vi "RSNRPZ Read Measurement.vi"(8 "error in (no error)":errorcluster, 9 "Timeout (5000 ms)":i32=5000, 10 "Channel (1)":i32=1, 11 "VISA session":refnum<visa-resource-name>) -> (0 "error out":errorcluster, 2 "Measurement":dbl format="%.3p", 3 "dup VISA session":refnum<visa-resource-name>)   [LabVIEW 2014]
doc: "This VI initiates an acquisition on the channels that you specifies in channel parameter. It then waits for the acquisition to complete, and returns the measurement for the channel you specify."
uses:
  rsnrpz_32.dll
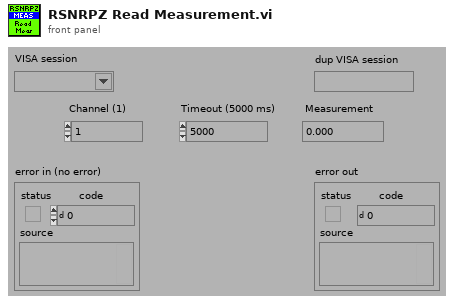
[diagram p1: front panel]
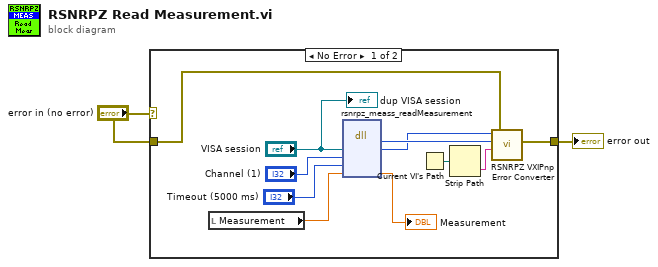
[diagram p0: block diagram]
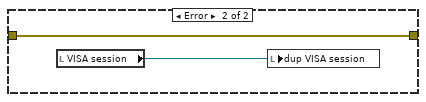
[diagram p2: hidden frame]
diagram:
  n1 = case shown="No Error" "error in (no error)" {
    tunnel: "error in (no error)" -> [w5 w15]
    tunnel: [w6 w15] -> w1
    frame No Error {
      n2 = local read "Measurement"() -> (w9:dbl)
      n3 = dll-call lib="rsnrpz_32.dll" fn="rsnrpz_meass_readMeasurement"("Instrument Handle"="VISA session", "Channel"="Channel (1)", "Timeout (ms)"="Timeout (5000 ms)", "Measurement"=w9) -> ("Status"=w12:i32, "Instrument Handle"=w7:u32, "Measurement"=→"Measurement":dbl)  [unwired: 5 in, 2 out]
      n4 = Current VI's Path() -> (path=w4:path)
      n5 = Strip Path(path=w4) -> (name=w3:string)  [unwired: 1 out]
      n6 = call "RSNRPZ VXIPnp Error Converter.vi"("error in (no error)"=w5, "name of VI"=w3, "VXIPnp error code"=w12, "VISA session"=w7) -> ("error out"=w6:errorcluster)  [unwired: 1 out]
      "dup VISA session" <- "VISA session"
    }
    frame Error {
      n7 = local read "VISA session"() -> (w14:refnum<visa-resource-name>)
      n8 = local write "dup VISA session"(w14) -> ()
    }
  }
  "error out" <- w1
